vi "Generate funct acq folder.vi"(8 "error in (no error)":errorcluster, 11 "Function":enum16{"Generate", "Obtain"}(ring)=enum."Obtain") -> (0 "error out":errorcluster, 3 "Funct acq experiment folder path":path)   [LabVIEW 2020]
uses:
  Logging/Typedefs/Experiment folder base name.ctl
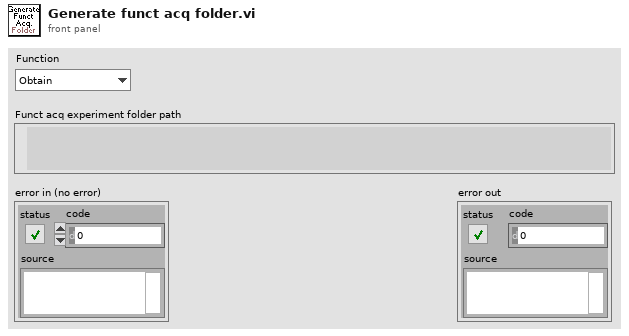
[diagram p1: front panel]
types:
  T1 = typedef "Experiment folder base name.ctl" = enum16{"TimeLapse", "FunctAcq"}
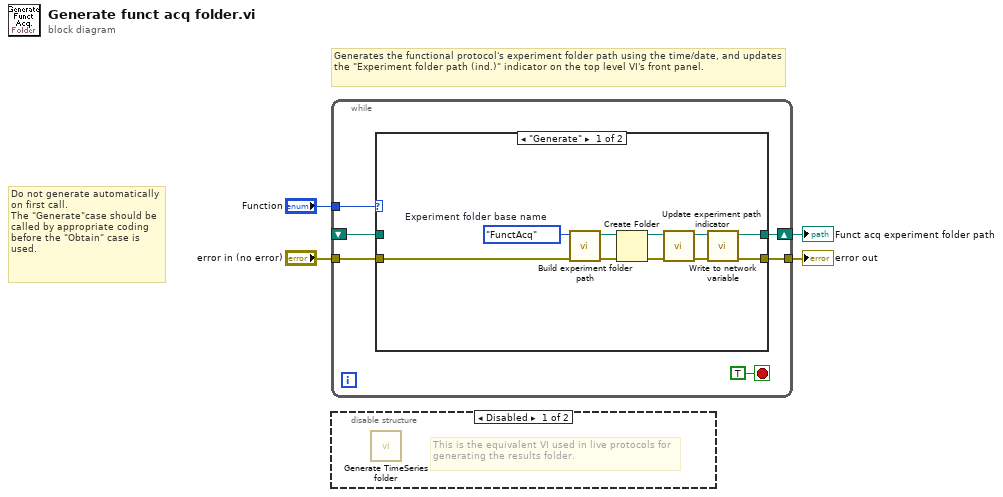
[diagram p0: block diagram]
diagram:
  # "Do not generate automatically on first call.\nThe \"Generate\"case should be called by appropriate coding before the \"Obtain\" case is used."
  # "Generates the functional protocol's experiment folder path using the time/date, and updates the \"Experiment folder path (ind.)\" indicator on the top level VI's front panel."
  n1 = while {
    tunnel: "error in (no error)" -> [w10]
    tunnel: [w8] -> w2
    shift-right: [w9] -> w3
    shift-left: _ -> [w6]
    tunnel: "Function" -> [w5]
    stop <- TRUE stop-if-true
    n2 = case shown="\"Generate\"" w5 {
      tunnel: w10 -> [w11 w21]
      tunnel: [w15 w22] -> w9
      tunnel: [w13 w21] -> w8
      tunnel: w6 -> [_ w22]
      frame "Generate" {
        w12 = Experiment_folder_base_name."FunctAcq"  # Experiment folder base name
        n3 = call "Build experiment folder path.vi"("error in (no error)"=w11, "Experiment folder base name"=w12) -> ("error out"=w19:errorcluster, "Experiment folder  file path"=w20:path)  [unwired: 8 in]
        n4 = Create Folder(path (use dialog)=w20, error in=w19) -> (created path=w17:path, error out=w18:errorcluster)  [unwired: 1 in, 1 out]
        n5 = call "Update experiment path indicator.vi"("error in (no error)"=w18, "created path"=w17) -> ("error out"=w14:errorcluster, "created path (dup)"=w16:path)  [unwired: 8 in]
        n6 = call "Write to network variable.vi"("error in (no error)"=w14, "created path"=w16) -> ("error out"=w13:errorcluster, "created path (dup)"=w15:path)  [unwired: 8 in]
      }
      frame "Obtain", Default {
      }
    }
  }
  "Funct acq experiment folder path" <- w3
  "error out" <- w2
  n7 = disable-structure shown="Disabled" {
    frame Disabled {
      # "This is the equivalent VI used in live protocols for generating the results folder."
      n8 = call "Generate TimeSeries folder.vi"() -> ()  [unwired: 10 in, 2 out]
    }
    frame Enabled {
    }
  }
